vi "探头通信分支.vi"(8 "探头属性":T3={"探头地址与信息"={"网络地址"={"IP"="10.10.100.254", "port"=8899}, "探头信息"="四渡赤水"}, "测量值"={"时间"=timestamp(0 s since 1904-01-01), "数值"=0.0}, "限值"={"限值1"=1.0, "限值2"=100.0}, "探头状态"=enum."离线"}, 11 "连接 ID":refnum<k5>) -> ()   [LabVIEW 2013]
doc: "独立的探头TCP连接的接收处理模块，具有\"创建TCP连接\"，“自动同步报警限值”，“掉线重连”，“解析实时数据与报警数据”的功能。"
uses:
  <vilib>/Platform/TimedLoop/XDataNode/XDataNode.xnode
  <vilib>/Platform/TimedLoop/XDataNode/nitl_modes.ctl
  <vilib>/Platform/TimedLoop/XDataNode/XDNodeRunTimeDep.lvlib
  <vilib>/Platform/TimedLoop/XDataNode/wakeup.ctl
  <vilib>/Platform/TimedLoop/XDataNode/timing_clust.ctl
panel:
  out "读数据":string
  out "循环次数":i32
  in  "通信错误":errorcluster caption="错误输出"
  in  "缓存结果":T1
  in  "改动项":T2={"探头信息"="", "启用？"=FALSE, "改动项"=enum."未改动", "限值"={"限值1"=1.0, "限值2"=100.0}}
  in  "停止":bool
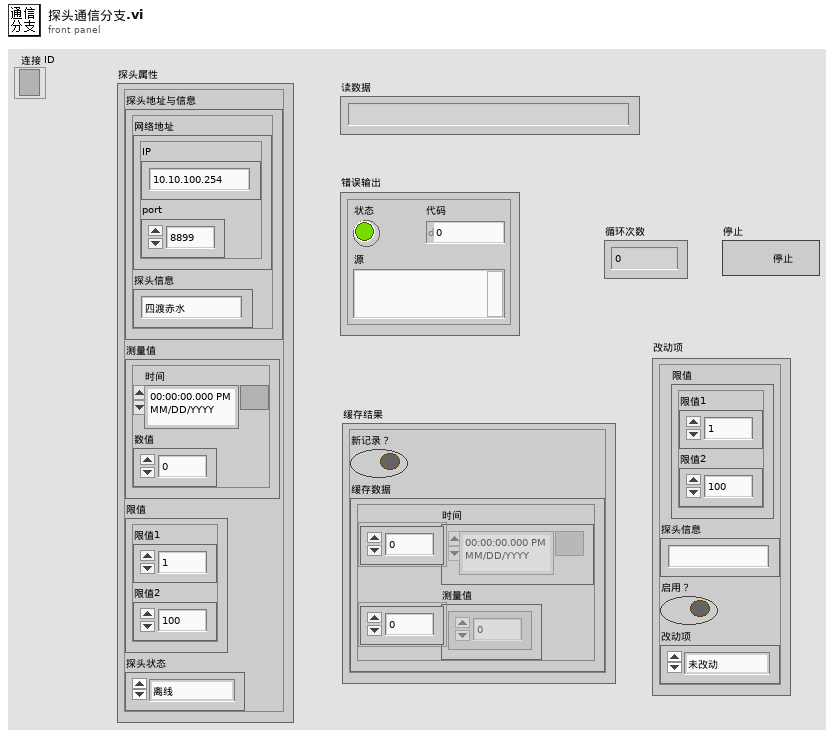
[diagram p1: front panel]
types:
  T1 = cluster{"新记录？":bool, "缓存数据":cluster{"时间":timestamp[], "测量值":dbl[]}}
  T2 = cluster{"探头信息":string, "启用？":bool, "改动项":enum16{"未改动", "改动-探头信息", "改动-启用状态", "改动-限值"}, "限值":cluster{"限值1":dbl, "限值2":dbl}}
  T3 = cluster{"探头地址与信息":cluster{"网络地址":cluster{"IP":string, "port":u16}, "探头信息":string}, "测量值":cluster{"时间":timestamp, "数值":dbl}, "限值":cluster{"限值1":dbl, "限值2":dbl}, "探头状态":enum16{"正常", "离线", "禁用", "一级报警", "二级报警"}}
  T4 = cluster{"探头信息":string, "启用？":bool, "改动项":enum16{"未改动", "改动-探头信息", "改动-启用状态"}}
  T5 = cluster{"网络地址":cluster{"IP":string, "port":u16}, "探头信息":string}
  T6 = enum16{"Standard", "Buffered", "CRLF", "Immediate"}
  T7 = cluster{"新记录？":bool, "实时缓存":cluster{"时间":timestamp[], "测量值":dbl[]}}
  T8 = typedef "XDNodeRunTimeDep.lvlib/timing_clust.ctl" = cluster{"Expected End [f-1]":u64, "Actual End [f-1]":u64, "Finished Late? [f-1]":bool, "Expected End [i-1]":u64, "Actual End [i-1]":u64, "Finished Late? [i-1]":bool, "Expected Start [i]":u64, "Actual Start [i]":u64, "Expected Start [f]":u64, "Actual Start [f]":u64, "Source Name":string, "Structure Name":string, "Period":i64, "Deadline":i64, "Offset":i64, "Start":i64, "Priority":i32, "Timeout":i32, "Mode":T9, "Wakeup Reason":T10, "Error":errorcluster, "Source Type":string, "Secondary Source Type":string, "Global End Time":u64, "Global Start Time":u64, "Frame Duration":u64, "Iteration Duration":u64, "Assigned CPU":i32, "I/O Scan Engine Mode":u32}
  T9 = typedef "XDNodeRunTimeDep.lvlib/nitl_modes.ctl" = enum32{"No Change", "Process missed periods, maintain original phase", "Discard missed periods, maintain original phase", "Process missed periods, ignore original phase", "Discard missed periods, ignore original phase"}
  T10 = typedef "XDNodeRunTimeDep.lvlib/wakeup.ctl" = enum32{"Normal", "Aborted", "Asynchronous wakeup", "Timing source error", "Timed loop error", "Timeout"}
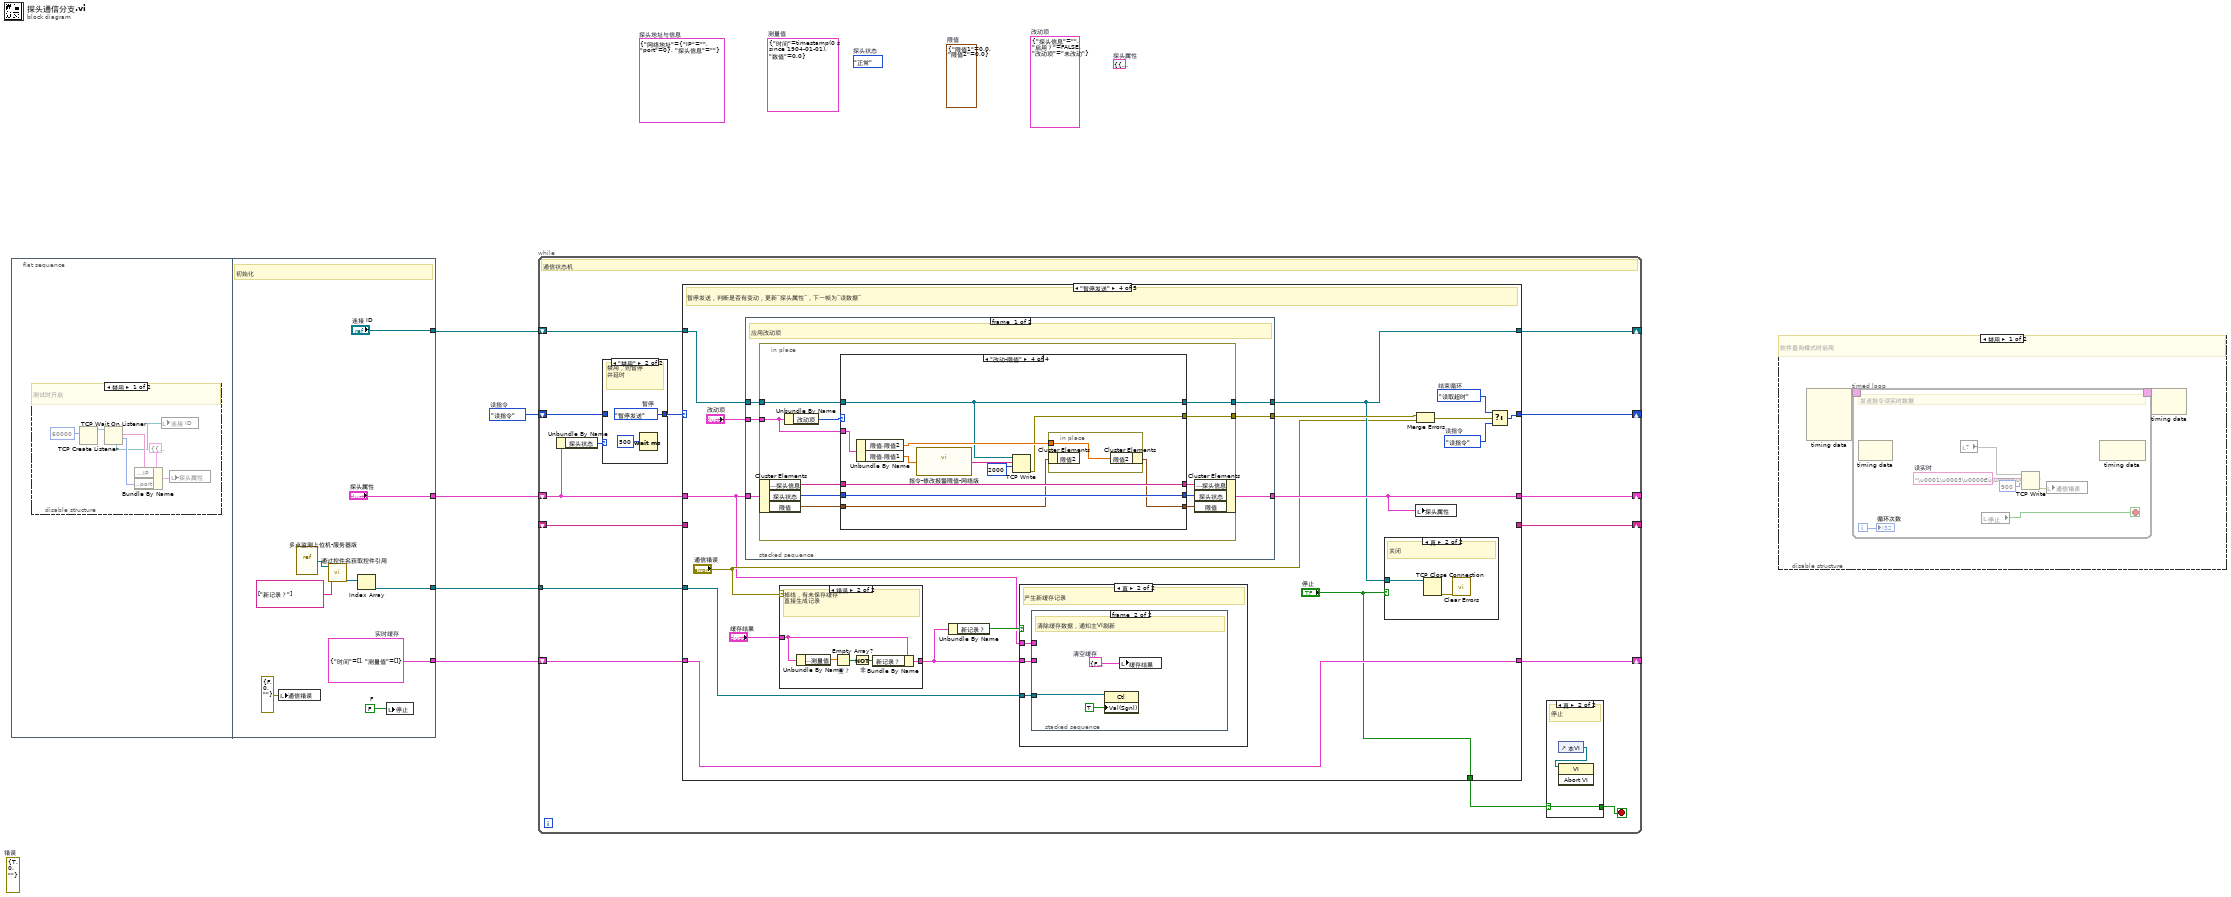
[diagram p0: block diagram]
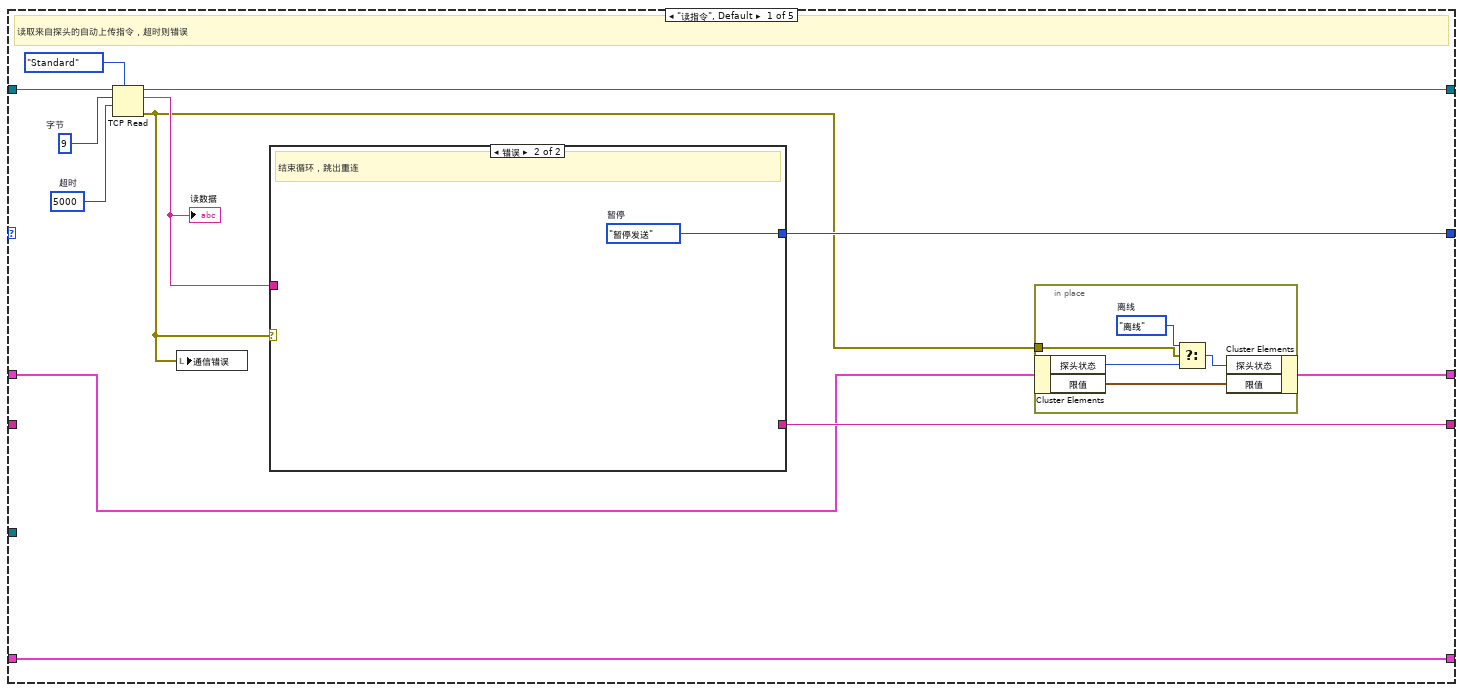
[diagram p5: hidden frame]
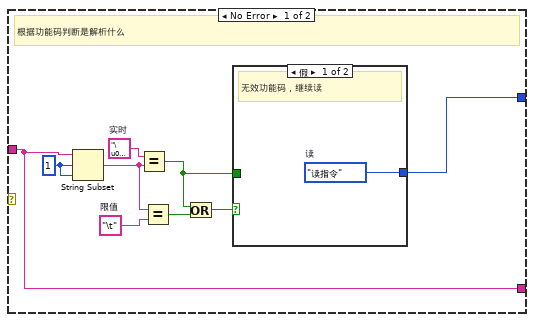
[diagram p6: hidden frame]
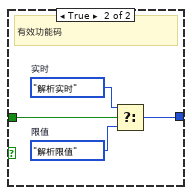
[diagram p7: hidden frame]
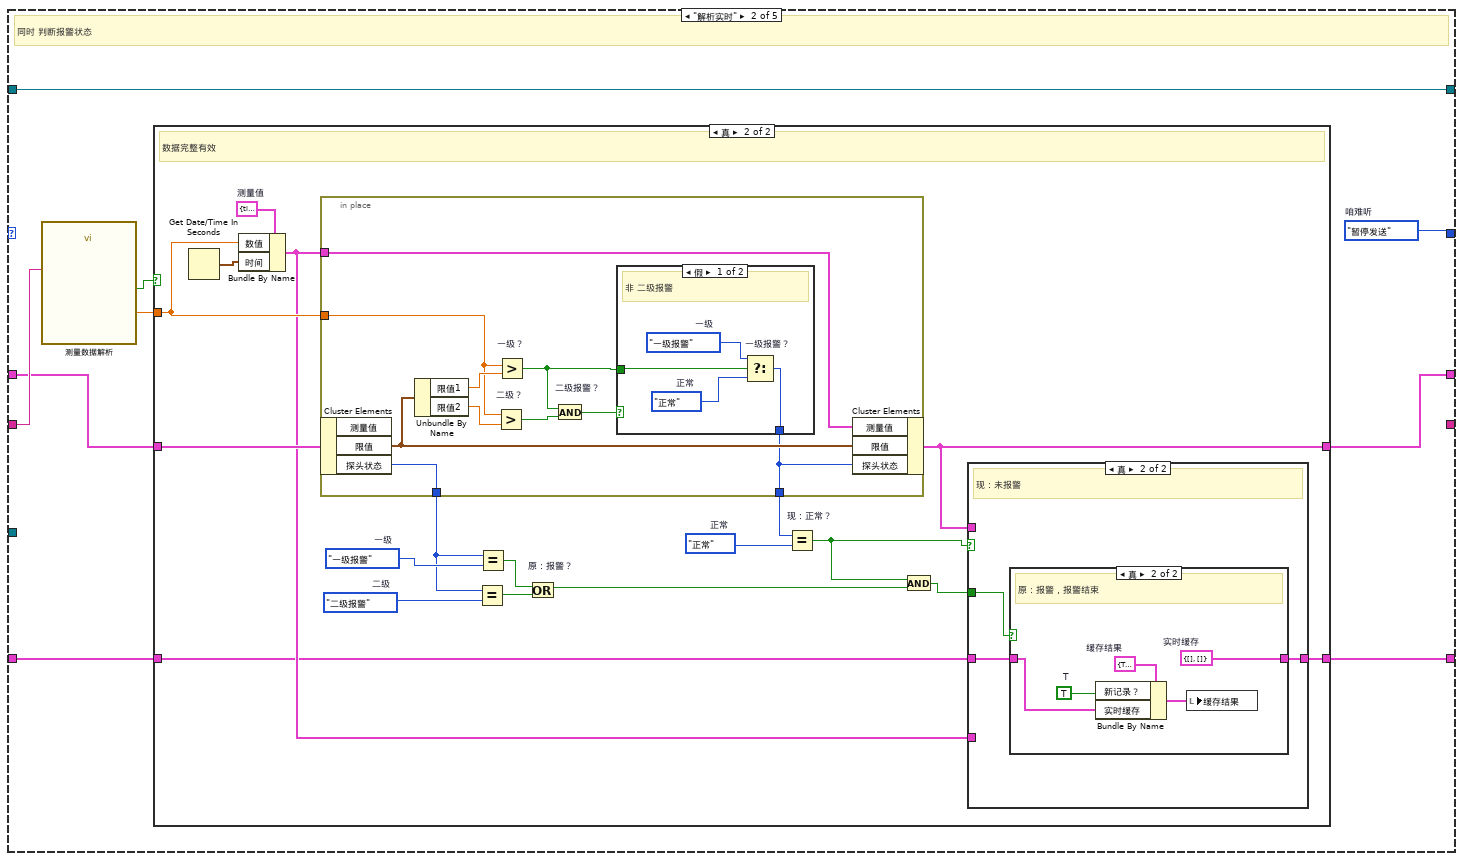
[diagram p8: hidden frame]
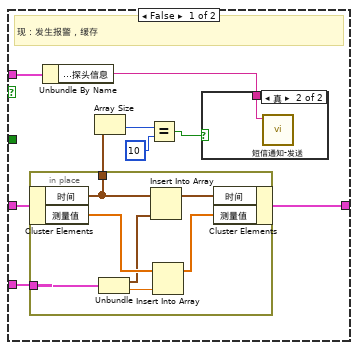
[diagram p10: hidden frame]
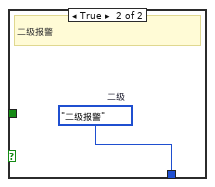
[diagram p13: hidden frame]
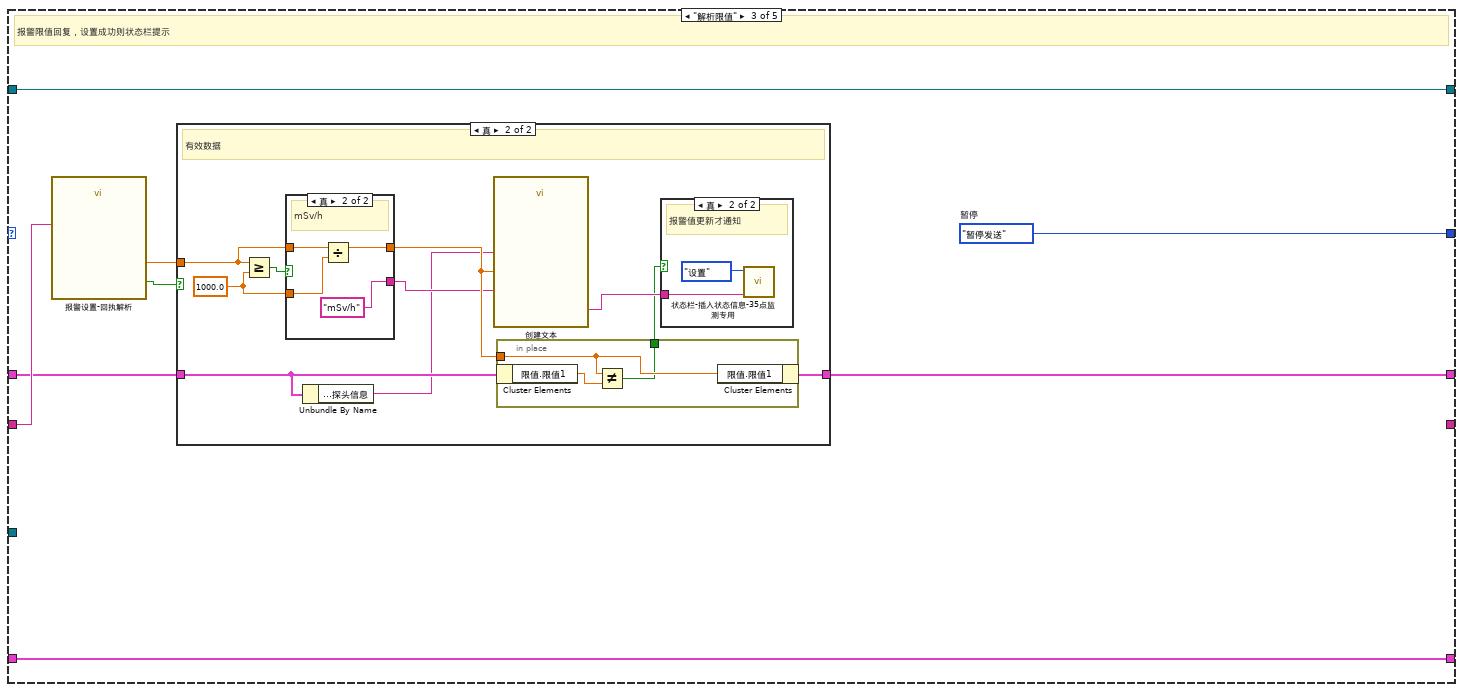
[diagram p14: hidden frame]
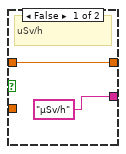
[diagram p17: hidden frame]
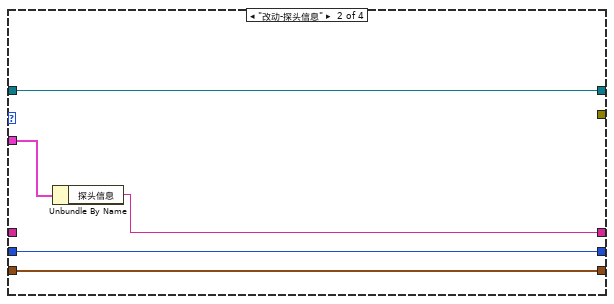
[diagram p20: hidden frame]
diagram:
  w4 = enum16{"读指令", "解析实时", "解析限值", "暂停发送", "读取超时"}."读指令"  # 读指令
  (unwired) T4 {"探头信息"="", "启用？"=FALSE, "改动项"=enum."未改动"}  # 改动项
  (unwired) T3 {"探头地址与信息"={"网络地址"={"IP"="", "port"=0}, "探头信息"=""}, "测量值"={"时间"=timestamp(0 s since 1904-01-01), "数值"=0.0}, "限值"={"限值1"=0.0, "限值2"=0.0}, "探头状态"=enum."正常"}  # 探头属性
  (unwired) errorcluster {"status"=TRUE, "code"=0, "source"=""}  # 错误
  (unwired) T5 {"网络地址"={"IP"="", "port"=0}, "探头信息"=""}  # 探头地址与信息
  (unwired) enum16{"正常", "离线", "禁用", "一级报警", "二级报警"}."正常"  # 探头状态
  (unwired) cluster{"限值1":dbl, "限值2":dbl} {"限值1"=0.0, "限值2"=0.0}  # 限值
  (unwired) cluster{"时间":timestamp, "数值":dbl} {"时间"=timestamp(0 s since 1904-01-01), "数值"=0.0}  # 测量值
  n1 = flat-sequence {
    tunnel: ["探头属性"] -> w3
    tunnel: [w20] -> w2
    tunnel: [w15] -> w5
    tunnel: ["连接 ID"] -> w1
    frame #0 {
      n2 = disable-structure shown="禁用" {
        frame Disabled {
          # "测试时开启"
          n3 = TCP Create Listener(10:u16 60000 ("端口")) -> (3:w12:refnum<k5>)  [unwired: 4 in, 2 out]
          n4 = TCP Wait On Listener(11:w12) -> (1:w8:u16, 2:w9:string, 4:w6:refnum<k5>)  [unwired: 3 in, 2 out]
          n5 = Bundle By Name(cluster=T3 {"探头地址与信息"={"网络地址"={"IP"="10.10.100.254", "port"=8899}, "探头信息"="四渡赤水"}, "测量值"={"时间"=timestamp(0 s since 1904-01-01), "数值"=0.0}, "限值"={"限值1"=1.0, "限值2"=100.0}, "探头状态"=enum."离线"} ("探头属性"), "探头地址与信息.网络地址.IP"=w9, "探头地址与信息.网络地址.port"=w8) -> (w7:T3)
          n6 = local write "连接 ID"(w6) -> ()
          n7 = local write "探头属性"(w7) -> ()
        }
        frame Enabled {
        }
      }
    }
    frame #1 {
      w19 = FALSE  # F
      w20 = cluster{"时间":timestamp[], "测量值":dbl[]} {"时间"=[], "测量值"=[]}  # 实时缓存
      # "初始化"
      n8 = local write "通信错误"(errorcluster {"status"=FALSE, "code"=0, "source"=""} ("通信错误")) -> ()
      n9 = vi-ref "多点监测上位机-服务器版.vi"() -> (w18:refnum<vi>)
      n10 = call "通过控件名获取控件引用.vi"("控件名数组"=string[] ["新记录？"], "VI引用"=w18) -> ("控件引用输出"=w16:refnum<vi>[])  [unwired: 7 in, 2 out]
      n11 = Index Array(array=w16) -> (element=w15:refnum<vi>)  [unwired: 1 in]
      n12 = local write "停止"(w19) -> ()
    }
  }
  n13 = while {
    shift-right: [w34] -> _
    shift-left: w4 -> [w27]
    shift-right: [w35] -> _
    shift-left: w1 -> [w36]
    shift-right: [w33] -> _
    shift-left: _ -> [w32]
    shift-right: [w31] -> _
    shift-left: w3 -> [w30]
    shift-right: [w26] -> _
    shift-left: w2 -> [w25]
    tunnel: w5 -> [w24]
    stop <- w22 stop-if-true
    # "通信状态机"
    n14 = Unbundle By Name(w30) -> ("探头状态"=w29:enum16{"正常", "离线", "禁用", "一级报警", "二级报警"})
    n15 = case shown="\"禁用\"" w29 {
      tunnel: [w40 w42] -> w28
      tunnel: w27 -> [w40 _]
      frame "正常", Default {
        # "启用，正常通过"
      }
      frame "禁用" {
        w42 = enum16{"读指令", "解析实时", "解析限值", "暂停发送", "读取超时"}."暂停发送"  # 暂停
        # "禁用，则暂停\n并延时"
        n16 = Wait (ms)(milliseconds to wait=u32 500 ("等待时间（毫秒）")) -> ()  [unwired: 1 out]
      }
    }
    n17 = case shown="\"暂停发送\"" w28 {
      tunnel: w36 -> [w54 w79 w148 w184 w273]
      tunnel: [w51 w79 w148 w181 w272] -> w35
      tunnel: [w49 w80 w149 w186 w275] -> w34
      tunnel: [_ _ _ "停止" w276] -> w23
      tunnel: [w48 _ _ _ _] -> w33
      tunnel: w32 -> [_ w83 w152 _ _]
      tunnel: w30 -> [w47 w78 w147 w177 w271]
      tunnel: [w46 w77 w146 w190 w271] -> w31
      tunnel: [w45 w76 w145 w185 w274] -> w26
      tunnel: w25 -> [w45 w75 w145 w185 w274]
      tunnel: w24 -> [_ _ _ w179 _]
      frame "读指令", Default {
        w52 = 5000  # 超时
        w53 = 9  # 字节
        # "读取来自探头的自动上传指令，超时则错误"
        n18 = TCP Read(connection ID=w54, bytes to read=w53, 7:T6."Standard" ("模式（标准）"), 9:w52) -> (connection ID out=w51:refnum<k5>, data out=w50:string, error out=w44:errorcluster)  [unwired: 1 in]
        "读数据" <- w50
        n19 = local write "通信错误"(w44) -> ()
        n20 = case shown="错误" w44 {
          tunnel: w50 -> [w60 _]
          tunnel: [w62 w74] -> w49
          tunnel: [w60 _] -> w48
          frame No Error {
            w66 = "\t"  # 限值
            w67 = "\u0003"  # 实时
            w68 = 1 ("偏移量(0)")
            # "根据功能码判断是解析什么"
            n21 = String Subset(string=w60, offset (0)=w68, length (rest)=w68) -> (substring=w65:string)
            n22 = Equal?(x=w67, y=w65) -> (x = y?=w61:bool)
            n23 = Equal?(x=w65, y=w66) -> (x = y?=w64:bool)
            n24 = Or(x=w61, y=w64) -> (x .or. y?=w63:bool)
            n25 = case shown="假" w63 {
              tunnel: [w69 w70] -> w62
              tunnel: w61 -> [_ w73]
              frame False {
                w69 = enum16{"读指令", "解析实时", "解析限值", "暂停发送", "读取超时"}."读指令"  # 读
                # "无效功能码，继续读"
              }
              frame True {
                w71 = enum16{"读指令", "解析实时", "解析限值", "暂停发送", "读取超时"}."解析限值"  # 限值
                w72 = enum16{"读指令", "解析实时", "解析限值", "暂停发送", "读取超时"}."解析实时"  # 实时
                # "有效功能码"
                n26 = Select(t=w72, s=w73, f=w71) -> (s? t:f=w70:enum16{"读指令", "解析实时", "解析限值", "暂停发送", "读取超时"})
              }
            }
          }
          frame Error {
            w74 = enum16{"读指令", "解析实时", "解析限值", "暂停发送", "读取超时"}."暂停发送"  # 暂停
            # "结束循环，跳出重连"
          }
        }
        n27 = in-place {
          in-place-border: w44 -> [w58]
          w57 = enum16{"正常", "离线", "禁用", "一级报警", "二级报警"}."离线"  # 离线
          n28 = in-place-cluster #1(w47) -> ("探头状态"=w55:enum16{"正常", "离线", "禁用", "一级报警", "二级报警"}, "限值"=w59:cluster{"限值1":dbl, "限值2":dbl})
          n29 = Select(t=w57, s=w58, f=w55) -> (s? t:f=w56:enum16{"正常", "离线", "禁用", "一级报警", "二级报警"})
          n30 = in-place-cluster #1("探头状态"=w56, "限值"=w59) -> (w46:T3)
        }
      }
      frame "解析实时" {
        w80 = enum16{"读指令", "解析实时", "解析限值", "暂停发送", "读取超时"}."暂停发送"  # 咱难听
        # "同时 判断报警状态"
        n31 = call "测量数据解析.vi"("完整输入"=w83) -> ("CRC？"=w82:bool, "测量值"=w81:dbl)  [unwired: 8 in, 1 out]
        n32 = case shown="真" w82 {
          tunnel: w81 -> [_ w100]
          tunnel: w78 -> [w85 w101]
          tunnel: [w85 w86] -> w77
          tunnel: [w84 w88] -> w76
          tunnel: w75 -> [w84 w87]
          frame False {
            # "数据不完整"
          }
          frame True {
            w97 = enum16{"正常", "离线", "禁用", "一级报警", "二级报警"}."一级报警"  # 一级
            w95 = enum16{"正常", "离线", "禁用", "一级报警", "二级报警"}."二级报警"  # 二级
            w98 = enum16{"正常", "离线", "禁用", "一级报警", "二级报警"}."正常"  # 正常
            w103 = cluster{"时间":timestamp, "数值":dbl} {"时间"=timestamp(0 s since 1904-01-01), "数值"=0.0}  # 测量值
            # "数据完整有效"
            n33 = Get Date/Time In Seconds() -> (seconds since 1Jan1904=w102:timestamp)
            n34 = Bundle By Name(cluster=w103, "数值"=w100, "时间"=w102) -> (w89:cluster{"时间":timestamp, "数值":dbl})
            n35 = in-place {
              in-place-border: w89 -> [w139]
              in-place-border: w100 -> [w136]
              in-place-border: [w131] -> w96
              in-place-border: [w130] -> w99
              n36 = in-place-cluster #2(w101) -> ("限值"=w138:cluster{"限值1":dbl, "限值2":dbl}, "探头状态"=w131:enum16{"正常", "离线", "禁用", "一级报警", "二级报警"})  [unwired: 1 out]
              n37 = Unbundle By Name(w138) -> ("限值1"=w137:dbl, "限值2"=w135:dbl)
              n38 = Greater? "二级？"(x=w136, y=w135) -> (0:w134:bool)
              n39 = Greater? "一级？"(x=w136, y=w137) -> (0:w133:bool)
              n40 = And "二级报警？"(x=w133, y=w134) -> (x .and. y?=w132:bool)
              n41 = case shown="假" w132 {
                tunnel: w133 -> [w143 _]
                tunnel: [w140 w144] -> w130
                frame False {
                  w142 = enum16{"正常", "离线", "禁用", "一级报警", "二级报警"}."正常"  # 正常
                  w141 = enum16{"正常", "离线", "禁用", "一级报警", "二级报警"}."一级报警"  # 一级
                  # "非 二级报警"
                  n42 = Select "一级报警？"(t=w141, s=w143, f=w142) -> (s? t:f=w140:enum16{"正常", "离线", "禁用", "一级报警", "二级报警"})
                }
                frame True {
                  w144 = enum16{"正常", "离线", "禁用", "一级报警", "二级报警"}."二级报警"  # 二级
                  # "二级报警"
                }
              }
              n43 = in-place-cluster #2("测量值"=w139, "限值"=w138, "探头状态"=w130) -> (w86:T3)
            }
            n44 = Equal?(x=w96, y=w95) -> (x = y?=w93:bool)
            n45 = Equal?(x=w96, y=w97) -> (x = y?=w94:bool)
            n46 = Or "原：报警？"(x=w94, y=w93) -> (x .or. y?=w92:bool)
            n47 = Equal? "现：正常？"(x=w99, y=w98) -> (x = y?=w91:bool)
            n48 = And(x=w91, y=w92) -> (x .and. y?=w90:bool)
            n49 = case shown="真" w91 {
              tunnel: w90 -> [_ w123]
              tunnel: w89 -> [w112 _]
              tunnel: w87 -> [w111 w121]
              tunnel: [w110 w122] -> w88
              tunnel: w86 -> [w106 _]
              frame False {
                # "现：发生报警，缓存"
                n50 = in-place {
                  in-place-border: w112 -> [w119]
                  in-place-border: [w114] -> w109
                  n51 = in-place-cluster #3(w111) -> ("时间"=w114:timestamp[], "测量值"=w120:dbl[])
                  n52 = Unbundle(w119) -> ("时间"=w118:timestamp, "数值"=w117:dbl)
                  n53 = Insert Into Array(array=w114, new element=w118) -> (w116:timestamp[])  [unwired: 1 in]
                  n54 = Insert Into Array(array=w120, new element=w117) -> (w115:dbl[])  [unwired: 1 in]
                  n55 = in-place-cluster #3("时间"=w116, "测量值"=w115) -> (w110:cluster{"时间":timestamp[], "测量值":dbl[]})
                }
                n56 = Unbundle By Name(w106) -> ("探头地址与信息.探头信息"=w105:string)
                n57 = Array Size(array=w109) -> (size(s)=w108:i32)
                n58 = Equal?(x=w108, y=10 ("x")) -> (x = y?=w104:bool)
                n59 = case shown="真" w104 {
                  tunnel: w105 -> [_ w113]
                  frame False {
                  }
                  frame True {
                    n60 = call "短信通知-发送.vi"("探头名称"=w113) -> ()  [unwired: 11 in]
                  }
                }
              }
              frame True {
                # "现：未报警"
                n61 = case shown="真" w123 {
                  tunnel: [w124 w129] -> w122
                  tunnel: w121 -> [w124 w126]
                  frame False {
                    # "原：未报警，正常"
                  }
                  frame True {
                    w128 = T7 {"新记录？"=TRUE, "实时缓存"={"时间"=[], "测量值"=[]}}  # 缓存结果
                    w127 = TRUE  # T
                    w129 = cluster{"时间":timestamp[], "测量值":dbl[]} {"时间"=[], "测量值"=[]}  # 实时缓存
                    # "原：报警，报警结束"
                    n62 = Bundle By Name(cluster=w128, "新记录？"=w127, "实时缓存"=w126) -> (w125:T7)
                    n63 = local write "缓存结果"(w125) -> ()
                  }
                }
              }
            }
          }
        }
      }
      frame "解析限值" {
        w149 = enum16{"读指令", "解析实时", "解析限值", "暂停发送", "读取超时"}."暂停发送"  # 暂停
        # "报警限值回复，设置成功则状态栏提示"
        n64 = call "报警设置-回执解析.vi"("完整输入"=w152) -> ("有效数据？"=w151:bool, "限值"=w150:dbl)  [unwired: 8 in, 1 out]
        n65 = case shown="真" w151 {
          tunnel: w150 -> [_ w162]
          tunnel: w147 -> [w153 w156]
          tunnel: [w153 w159] -> w146
          frame False {
            # "无效数据"
          }
          frame True {
            w161 = 1000.0 ("y")
            # "有效数据"
            n66 = Greater Or Equal?(x=w162, y=w161) -> (x >= y?=w163:bool)
            n67 = case shown="真" w163 {
              tunnel: [w170 w172] -> w158
              tunnel: w162 -> [w170 w173]
              tunnel: ["μSv/h" ("单位") "mSv/h" ("单位")] -> w157
              tunnel: w161 -> [_ w171]
              frame False {
                # "uSv/h"
              }
              frame True {
                # "mSv/h"
                n68 = Divide(x=w173, y=w171) -> (x/y=w172:dbl)
              }
            }
            n69 = Unbundle By Name(w156) -> ("探头地址与信息.探头信息"=w155:string)
            n70 = call "创建文本"("探头名称"=w155, "限值"=w158, "单位"=w157) -> ("Result"=w160:string)  [unwired: 11 in, 1 out]
            n71 = in-place {
              in-place-border: w158 -> [w167]
              in-place-border: [w166] -> w154
              n72 = in-place-cluster #4(w156) -> ("限值.限值1"=w168:dbl)
              n73 = Not Equal?(x=w167, y=w168) -> (x != y?=w166:bool)
              n74 = in-place-cluster #4("限值.限值1"=w167) -> (w159:T3)
            }
            n75 = case shown="真" w154 {
              tunnel: w160 -> [_ w164]
              frame False {
              }
              frame True {
                # "报警值更新才通知"
                n76 = call "状态栏-插入状态信息-35点监测专用.vi"("消息内容"=w164, "状态类型"=enum16{"全部", "报警", "通信", "设置"}."设置") -> ()  [unwired: 10 in]
              }
            }
          }
        }
      }
      frame "暂停发送" {
        w188 = enum16{"读指令", "解析实时", "解析限值", "暂停发送", "读取超时"}."读取超时"  # 结束循环
        w187 = enum16{"读指令", "解析实时", "解析限值", "暂停发送", "读取超时"}."读指令"  # 读指令
        # "暂停发送，判断是否有变动，更新“探头属性”，下一帧为“读数据”"
        n77 = stacked-sequence {
          tunnel: "改动项" -> [w203 _]
          tunnel: [w202 _] -> w190
          tunnel: w177 -> [w201 _]
          tunnel: w184 -> [w200 _]
          tunnel: [w199 _] -> w183
          tunnel: [w198 _] -> w181
          frame #0 {
            # "应用改动项"
            n78 = in-place {
              in-place-border: w203 -> [w213]
              in-place-border: w200 -> [w206]
              in-place-border: [w205] -> w198
              in-place-border: [w204] -> w199
              n79 = in-place-cluster #5(w201) -> ("探头地址与信息.探头信息"=w211:string, "探头状态"=w210:enum16{"正常", "离线", "禁用", "一级报警", "二级报警"}, "限值"=w208:cluster{"限值1":dbl, "限值2":dbl})
              n80 = Unbundle By Name(w213) -> ("改动项"=w214:enum16{"未改动", "改动-探头信息", "改动-启用状态", "改动-限值"})
              n81 = case shown="\"改动-限值\"" w214 {
                tunnel: w213 -> [_ w223 w233 w249]
                tunnel: [w218 w222 w229 w252] -> w212
                tunnel: w211 -> [w218 _ w229 w252]
                tunnel: [w217 w221 w228 w251] -> w209
                tunnel: w210 -> [w217 w221 _ w251]
                tunnel: w208 -> [w216 w220 w225 w250]
                tunnel: [w216 w220 w225 w247] -> w207
                tunnel: w206 -> [w215 w219 w227 w243]
                tunnel: [w215 w219 w226 w243] -> w205
                tunnel: [_ _ w224 w242] -> w204
                frame "未改动", Default {
                  # "未改动"
                }
                frame "改动-探头信息" {
                  n82 = Unbundle By Name(w223) -> ("探头信息"=w222:string)
                }
                frame "改动-启用状态" {
                  w231 = enum16{"正常", "离线", "禁用", "一级报警", "二级报警"}."禁用"  # 禁用
                  w230 = enum16{"正常", "离线", "禁用", "一级报警", "二级报警"}."正常"  # 正常
                  n83 = Unbundle By Name(w233) -> ("启用？"=w232:bool)
                  n84 = Select(t=w230, s=w232, f=w231) -> (s? t:f=w228:enum16{"正常", "离线", "禁用", "一级报警", "二级报警"})
                  n85 = case shown="\"正常\", 默认" w228 {
                    tunnel: w225 -> [w240 _]
                    tunnel: w227 -> [w236 w241]
                    tunnel: [w235 w241] -> w226
                    tunnel: [w234 _] -> w224
                    frame "正常", Default {
                      # "启用探头，同步报警值"
                      n86 = Unbundle By Name(w240) -> ("限值1"=w239:dbl)
                      n87 = call "指令-修改报警限值-网络版.vi"("限值1"=w239) -> ("指令输出"=w237:string)  [unwired: 10 in]
                      n88 = TCP Write(connection ID=w236, data in=w237, 9:2000 ("超时毫秒(25000)")) -> (connection ID out=w235:refnum<k5>, error out=w234:errorcluster)  [unwired: 1 in, 1 out]
                    }
                    frame "禁用" {
                    }
                  }
                }
                frame "改动-限值" {
                  n89 = Unbundle By Name(w249) -> ("限值.限值2"=w248:dbl, "限值.限值1"=w244:dbl)
                  n90 = call "指令-修改报警限值-网络版.vi"("限值1"=w244) -> ("指令输出"=w246:string)  [unwired: 10 in]
                  n91 = TCP Write(connection ID=w243, data in=w246, 9:2000 ("超时毫秒(25000)")) -> (error out=w242:errorcluster)  [unwired: 1 in, 2 out]
                  n92 = in-place {
                    in-place-border: w248 -> [w253]
                    n93 = in-place-cluster #6(w250) -> ()  [unwired: 1 out]
                    n94 = in-place-cluster #6("限值2"=w253) -> (w247:cluster{"限值1":dbl, "限值2":dbl})
                  }
                }
              }
              n95 = in-place-cluster #5("探头地址与信息.探头信息"=w212, "探头状态"=w209, "限值"=w207) -> (w202:T3)
            }
          }
          frame #1 {
            w254 = T2 {"探头信息"="", "启用？"=FALSE, "改动项"=enum."未改动", "限值"={"限值1"=1.0, "限值2"=100.0}}  # 改动项
            # "改动项复位"
            n96 = local write "改动项"(w254) -> ()
          }
        }
        n97 = case shown="错误" "通信错误" {
          tunnel: "缓存结果" -> [w192 w196]
          tunnel: [w192 w193] -> w175
          frame No Error {
            # "正常执行"
          }
          frame Error {
            # "掉线，有未保存缓存\n直接生成记录"
            n98 = Unbundle By Name(w196) -> ("缓存数据.测量值"=w197:dbl[])
            n99 = Empty Array? "空？"(array=w197) -> (empty?=w195:bool)
            n100 = Not "非"(x=w195) -> (.not. x?=w194:bool)
            n101 = Bundle By Name(cluster=w196, "新记录？"=w194) -> (w193:T1)
          }
        }
        n102 = Unbundle By Name(w175) -> ("新记录？"=w189:bool)
        n103 = case shown="真" w189 {
          tunnel: w175 -> [_ w259]
          tunnel: w177 -> [_ w258]
          tunnel: w179 -> [_ w257]
          frame False {
            # "没有新缓存"
          }
          frame True {
            # "产生新缓存记录"
            n104 = stacked-sequence {
              tunnel: w259 -> [w262 _]
              tunnel: w258 -> [w261 _]
              tunnel: w257 -> [_ w264]
              frame #0 {
                # "生成缓存文件"
                n105 = Unbundle By Name(w262) -> ("缓存数据"=w260:cluster{"时间":timestamp[], "测量值":dbl[]})
                n106 = call "生成-报警记录缓存数据文件-分类计时-网络版.vi"("缓存绘图数据"=w260, "探头属性"=w261) -> ()  [unwired: 10 in]
              }
              frame #1 {
                w265 = T1 {"新记录？"=FALSE, "缓存数据"={"时间"=[], "测量值"=[]}}  # 清空缓存
                # "清除缓存数据，通知主VI刷新"
                n107 = property class="Ctl"(reference=w264, "Val(Sgnl)"=TRUE) -> ()  [unwired: 1 in, 2 out]
                n108 = local write "缓存结果"(w265) -> ()
              }
            }
          }
        }
        n109 = case shown="真" "停止" {
          tunnel: w181 -> [_ w256]
          frame False {
          }
          frame True {
            # "关闭"
            n110 = TCP Close Connection(connection ID=w256) -> (error out=w255:errorcluster)  [unwired: 2 in, 1 out]
            n111 = call <vilib>:"Clear Errors.vi"("error in (no error)"=w255) -> ()  [unwired: 6 in, 1 out]
          }
        }
        n112 = local write "探头属性"(w190) -> ()
        n113 = Merge Errors(w183, "通信错误") -> (w182:errorcluster)
        n114 = Select(t=w188, s=w182, f=w187) -> (s? t:f=w186:enum16{"读指令", "解析实时", "解析限值", "暂停发送", "读取超时"})
      }
      frame "读取超时" {
        w275 = enum16{"读指令", "解析实时", "解析限值", "暂停发送", "读取超时"}."读指令"  # 读指令
        w276 = TRUE  # T
        # "关闭连接，结束循环，跳出重连"
        n115 = Unbundle By Name(w271) -> ("探头地址与信息.探头信息"=w270:string)
        n116 = TCP Close Connection(connection ID=w273, abort (F)=TRUE ("中止(F)")) -> (connection ID out=w272:refnum<k5>, error out=w268:errorcluster)  [unwired: 1 in]
        n117 = call "创建文本2"("探头名称"=w270) -> ("Result"=w269:string)  [unwired: 13 in, 1 out]
        n118 = call <vilib>:"Clear Errors.vi"("error in (no error)"=w268) -> ()  [unwired: 6 in, 1 out]
        n119 = call "状态栏-插入状态信息-35点监测专用.vi"("消息内容"=w269, "状态类型"=enum16{"全部", "报警", "通信", "设置"}."通信") -> ()  [unwired: 10 in]
      }
    }
    n120 = case shown="真" w23 {
      selector: w23 -> [w37 w38]
      tunnel: [w37 w38] -> w22
      frame False {
      }
      frame True {
        # "停止"
        n121 = control-ref of="本VI"() -> (w39:refnum<vi>)
        n122 = invoke class="VI" method="Abort VI"(reference=w39) -> ()  [unwired: 2 in, 3 out]
      }
    }
  }
  n123 = disable-structure shown="禁用" {
    frame Disabled {
      # "软件查询模式时启用"
      n124 = node-c288() -> (w278:T8)  [unwired: 4 in]
      n125 = timed-loop {
        timing: w278 -> [_]
        timing-out: [_] -> w277
        i -> [w280]
        stop <- w279 stop-if-true
        w282 = "\u0001\u0003\u0000€ú\u0000\u0006‚"  # 读实时
        # "发送指令读实时数据"
        n126 = node-c288() -> ()  [unwired: 1 in, 1 out]
        n127 = local read item#-1() -> (w283)
        n128 = local read "停止"() -> (w279:bool)
        n129 = TCP Write(connection ID=w283, data in=w282, 9:900 ("超时毫秒(25000)")) -> (error out=w281:errorcluster)  [unwired: 1 in, 2 out]
        n130 = local write "通信错误"(w281) -> ()
        n131 = node-c288() -> ()  [unwired: 1 in, 1 out]
        "循环次数" <- w280
      }
      n132 = node-c288(w277) -> ()  [unwired: 1 out]
    }
    frame Enabled {
    }
  }
